vi "LVDimInterface.dic_info_service_once.vi"(1 "serviceName":string, 3 "timeout [ms]":u32=10000, 5 "error in (no error)":errorcluster) -> (15 "data":i8[](array[numeric]), 16 "typeDescriptor":string, 17 "timed out?":bool, 19 "error out":errorcluster)   [LabVIEW 2015, in "LVDimInterface.lvlib"]
doc: "Obtains data of a service once. Important: For performance reasons, this VI should only be used, if one is interested in service data just once. \n\nHistory: 08-MAY-2006, Dietrich Beck\n\nCopyright (C)\nGesellschaft für Schwerionenforschung, GSI\nPlanckstr. 1\n64291 Darmstadt\nGermany\n\nContact: D.Beck@gsi.de \n\nThis program is free software; you can redistribute it and/or modify it under the terms of the \nGNU General Public License as published by the Free Software Foundation; either version 2 of the license, or (at your option) any later version.\n\nThis program is distributed in the hope that it will be useful, but WITHOUT ANY WARRANTY; without even the implied warranty of MERCHANTABILITY or FITNESS FOR A PARTICULAR PURPOSE. See the GNU General License for more details (http://www.gnu.org).\n\nGesellschaft für Schwerionenforschung, GSI\nPlanckstr. 1, 64291 Darmstadt, Germany\nFor all questions and ideas contact D. Beck.\nLast update: 16-DEC-2005"
uses:
  LVDimInterface.lvlib
  LVDimInterface.dim service type.ctl
  LVDimInterface.dic_info_service_notifier.vi
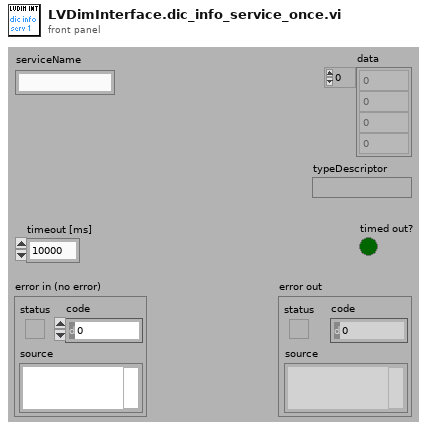
[diagram p1: front panel]
types:
  T1 = typedef "LVDimInterface.lvlib/LVDimInterface.dim service type.ctl" = u16
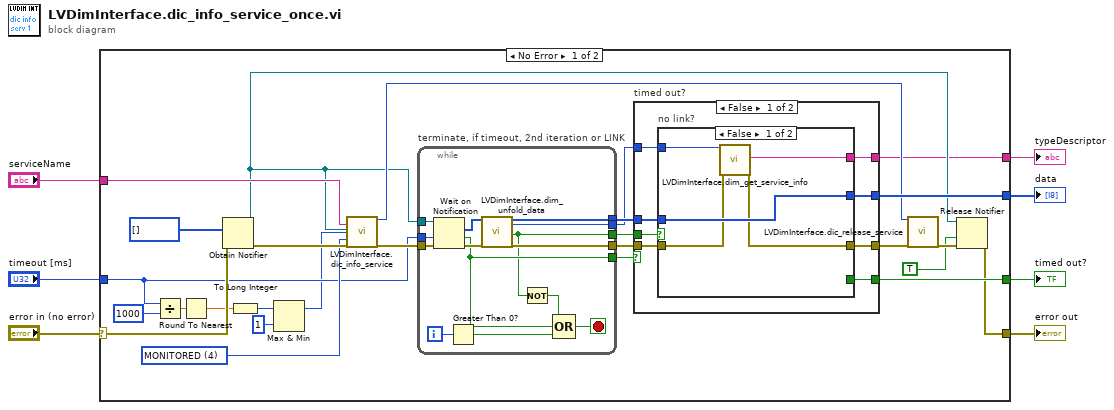
[diagram p0: block diagram]
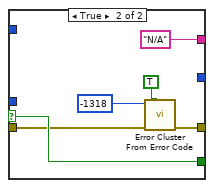
[diagram p2: hidden frame]
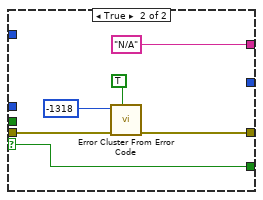
[diagram p3: hidden frame]
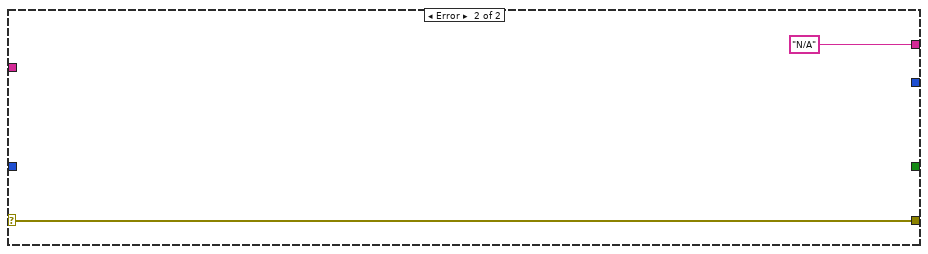
[diagram p4: hidden frame]
diagram:
  n1 = case shown="No Error" "error in (no error)" {
    selector: "error in (no error)" -> [w33 w75]
    tunnel: [w17 w75] -> w6
    tunnel: "serviceName" -> [w27 _]
    tunnel: "timeout [ms]" -> [w22 _]
    tunnel: [w28 _] -> w3
    tunnel: [w26 _] -> w2
    tunnel: [w16 "N/A" ("typeDescriptor")] -> w1
    frame No Error {
      w31 = T1 4 items=["ONCE_ONLY"=1, "TIMED"=2, "MONITORED"=4] ("serviceType")
      n2 = Divide(x=w22, y=1000) -> (x/y=w24:dbl)
      n3 = Round To Nearest(number=w24) -> (nearest integer value=w23:dbl)
      n4 = Obtain Notifier(notification data type=i8[] [], error in (no error)=w33) -> (notifier out=w18:refnum<notifier>, error out=w32:errorcluster)  [unwired: 2 in, 1 out]
      n5 = To Long Integer(number=w23) -> (32bit integer=w14:i32)
      n6 = Max & Min(x=w14, y=1) -> (max(x,y)=w12:i32)  [unwired: 1 out]
      n7 = call-poly "LVDimInterface.dic_info_service.vi"("serviceName"=w27, "notifierRef"=w18, "timeout [s]"=w12, "serviceType"=w31, "error in (no error)"=w32) -> ("callBackID"=w20:i32, "error out"=w30:errorcluster)  [unwired: 13 in]
      n8 = while "terminate, if timeout, 2nd iteration or LINK" {
        tunnel: w30 -> [w48]
        tunnel: [w39] -> w29
        tunnel: w22 -> [w47]
        tunnel: w18 -> [w46]
        tunnel: [w44] -> w11
        tunnel: [w42] -> w10
        tunnel: [w41] -> w9
        tunnel: [w38] -> w8
        i -> [w36]
        stop <- w40 stop-if-true
        n9 = Wait on Notification(notifier=w46, timeout in ms (-1)=w47, error in (no error)=w48) -> (notification=w43:i8[], timed out?=w39:bool, error out=w45:errorcluster)  [unwired: 1 in, 1 out]
        n10 = Greater Than 0?(x=w36) -> (x > 0?=w35:bool)
        n11 = call "LVDimInterface.dim_unfold_data.vi"("rawData"=w43, "error in (no error)"=w45) -> ("data"=w42:i8[], "callBackID"=w41:i32, "no link"=w38:bool, "error out"=w44:errorcluster)  [unwired: 14 in]
        n12 = Not(x=w38) -> (.not. x?=w37:bool)
        n13 = Compound Arithmetic op=OR(w37, w39, w35) -> (w40:bool)
      }
      n14 = case "timed out?" shown="False" w29 {
        selector: w29 -> [_ w73]
        tunnel: w11 -> [w49 w71]
        tunnel: [w56 _] -> w28
        tunnel: [w55 w73] -> w26
        tunnel: [w54 w70] -> w21
        tunnel: [w53 "N/A" ("typeDescriptor")] -> w16
        tunnel: w10 -> [w52 _]
        tunnel: w9 -> [w51 _]
        tunnel: w8 -> [w50 _]
        frame False {
          n15 = case "no link?" shown="False" w50 {
            selector: w50 -> [_ w67]
            tunnel: [w61 _] -> w56
            tunnel: w52 -> [w61 _]
            tunnel: [_ w67] -> w55
            tunnel: [w57 w64] -> w54
            tunnel: w49 -> [w58 w65]
            tunnel: [w59 "N/A" ("typeDescriptor")] -> w53
            tunnel: w51 -> [w60 _]
            frame False {
              n16 = call "LVDimInterface.dim_get_service_info.vi"("callBackID"=w60, "error in (no error)"=w58) -> ("typeDescriptor"=w59:string, "error out"=w57:errorcluster)  [unwired: 8 in, 8 out]
            }
            frame True {
              n17 = call <vilib>:"Error Cluster From Error Code.vi"("show call chain? (False)"=TRUE ("status"), "error in (no error)"=w65, "error code (0)"=-1318 ("code")) -> ("error out"=w64:errorcluster)  [unwired: 6 in]
            }
          }
        }
        frame True {
          n18 = call <vilib>:"Error Cluster From Error Code.vi"("show call chain? (False)"=TRUE ("status"), "error in (no error)"=w71, "error code (0)"=-1318 ("code")) -> ("error out"=w70:errorcluster)  [unwired: 6 in]
        }
      }
      n19 = call "LVDimInterface.dic_release_service.vi"("callBackID"=w20, "error in (no error)"=w21) -> ("error out"=w19:errorcluster)  [unwired: 17 in]
      n20 = Release Notifier(notifier=w18, force destroy? (F)=TRUE, error in (no error)=w19) -> (error out=w17:errorcluster)  [unwired: 2 out]
    }
    frame Error {
    }
  }
  "error out" <- w6
  "data" <- w3
  "timed out?" <- w2
  "typeDescriptor" <- w1
